vi "运维调试_五参数.vi"(11 "编号":string) -> ()   [LabVIEW 2016, in "斯坦道多参数.lvlib"]
uses:
  <vilib>/Utility/miscctls.llb/LVPointTypeDef.ctl
  <vilib>/Plasmionique/MB Master/MB_Master/MB_Master.lvclass
  <vilib>/Utility/config.llb/NI_LVConfig.lvlib
panel:
  in  "滤波次数":dbl caption="滤波次数:"
  in  "校准选择":T1
  out "模块版本号":string
  out "权限等级":string
  in  "ORP探头选择":u16(ring) items=["YL型", "MQ型", "NAQ型"]
  in  "ORP启用":bool
  in  "水样测量时间":dbl caption="水样测量时间:"
  in  "自动断线重连":bool=TRUE
  in  "打开modbus":bool
  out "选项卡控件":enum32{"选项卡 1", "选项卡 2"}(tab)
  in  "VISA资源名称":refnum<visa-resource-name> caption="串口"
  in  "IP":string="localhost" caption="IP:"
  in  "Port":u16=502 caption="Port:"
  in  "连接方式":u16(ring) items=["Modbus RTU", "Modbus TCP"]
  in  "密码锁":bool
  in  "藻密度探头选择":u16(ring) items=["YL型", "MQ型", "NAQ型"]
  in  "叶绿素a探头选择":u16(ring) items=["YL型", "MQ型", "NAQ型"]
  in  "浊度探头选择":u16(ring) items=["YL型", "MQ型", "NAQ型"]
  in  "电导率探头选择":u16(ring) items=["YL型", "MQ型", "NAQ型"]
  in  "DO探头选择":u16(ring) items=["YL型", "MQ型", "NAQ型"]
  in  "pH探头选择":u16(ring) items=["YL型", "MQ型", "NAQ型"]
  in  "设置页返回":bool
  in  "藻密度":bool
  in  "叶绿素a启用":bool
  in  "Temp":bool
  in  "Cond":bool
  in  "Turb":bool
  in  "DO":bool
  in  "pH":bool
  in  "周期设置":bool
  out "当前串口":string
  out "运行状态":enum16{"空闲", "水样测试", "标样核查"}(ring)
  in  "停止":bool
  in  "标样核查":bool
  in  "水样测试":bool
  in  "设置":bool
  in  "探头校正返回":bool
  in  "探头校正":bool
  out "检测值":T2
  # "请设置仪器连接方式"
  # "请选择要启用的参数"
  # "min"
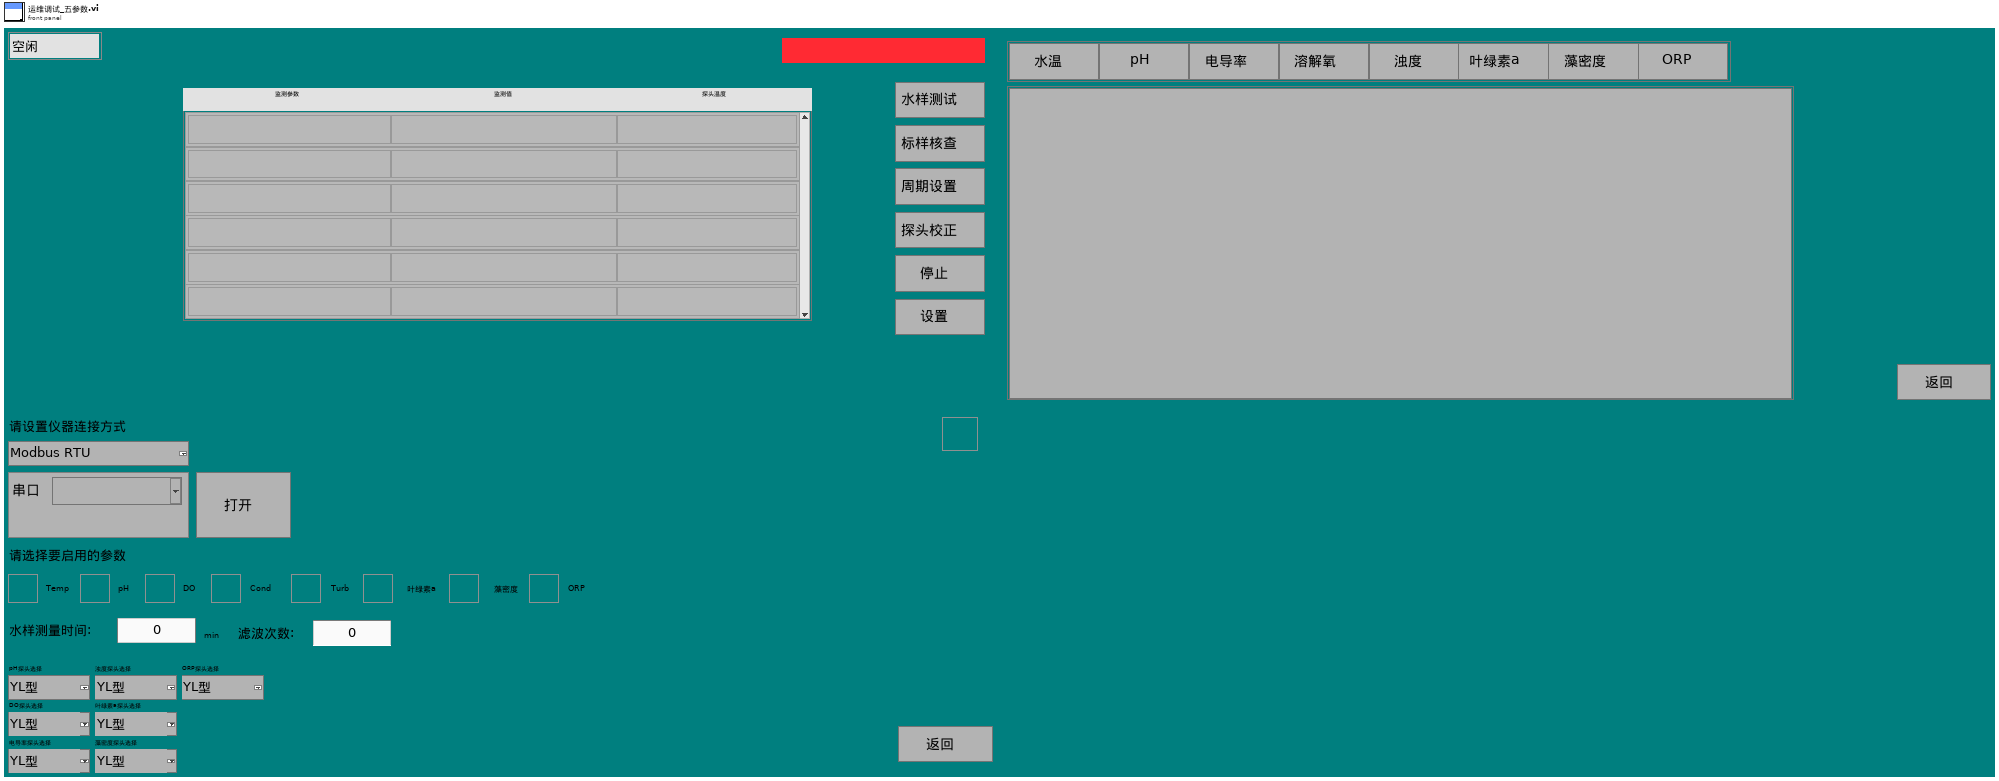
[diagram p1: front panel]
types:
  T1 = cluster{"水温校准":bool, "pH校准":bool, "电导率校准":bool, "溶解氧校准":bool, "浊度校准":bool, "叶绿素a校准":bool, "藻密度校准":bool, "ORP校准":bool}
  T2 = typedef "斯坦道多参数.lvlib/检测值.ctl" = cluster{"监测参数1":string, "浓度1":string, "探头温度1":string}[]
  T3 = typedef "LVPointTypeDef.ctl" = cluster{"Horizontal":i16, "Vertical":i16}
  T4 = enum8{"Enabled", "Disabled", "Disabled and Grayed Out"}
  T5 = cluster{"pH探头选择":u16, "DO探头选择":u16, "电导率探头选择":u16, "浊度探头选择":u16, "叶绿素a探头选择":u16, "蓝绿藻探头选择":u16, "orp探头选择":u16}
  T6 = cluster{"周期设置类型":enum16{"定点启动", "间隔启动"}, "定时功能启用":bool, "定时间隔":u32, "24H周期设置":bool[]}
  T7 = enum32{"Bad", "Idle", "Run top level", "Running"}
  T8 = typedef "LVDateTimeRec.ctl" = cluster{"秒数的小数部分":dbl, "秒":i32, "分":i32, "时":i32, "日":i32, "月":i32, "年":i32, "天数（周）":i32, "天数（年）":i32, "DST":i32}
  T9 = cluster{"Major":u16, "Minor":u16, "Fix":u16, "Build":u16}
  T10 = cluster{"监测参数1":string, "浓度1":string, "探头温度1":string}[]
  T11 = cluster{"温度测量值":sgl, "DO%":sgl, "DOmg/L":sgl, "温度偏移修正值":sgl}
  T12 = typedef "NI_LVConfig.lvlib/Config Data RefNum.ctl" = refnum<k1>
  T13 = cluster{"pH校准VI引用句柄":refnum<vi>, "DO校准VI引用句柄":refnum<vi>, "COND校准VI引用句柄":refnum<vi>, "TURB校准VI引用句柄":refnum<vi>, "CHLA校准VI引用句柄":refnum<vi>, "BGA校准VI引用句柄":refnum<vi>, "ORP校准VI引用句柄":refnum<vi>}
  T14 = cluster{"数据保存间隔":dbl, "水温标样值":dbl, "pH标样值":dbl, "溶解氧标样值":dbl, "电导率标样值":dbl, "浊度标样值":dbl}
  T15 = cluster{"baud rate (bps)":u32, "stop bits":u16, "parity":u16, "flow control":u16, "timeout":u32, "retries":i32}
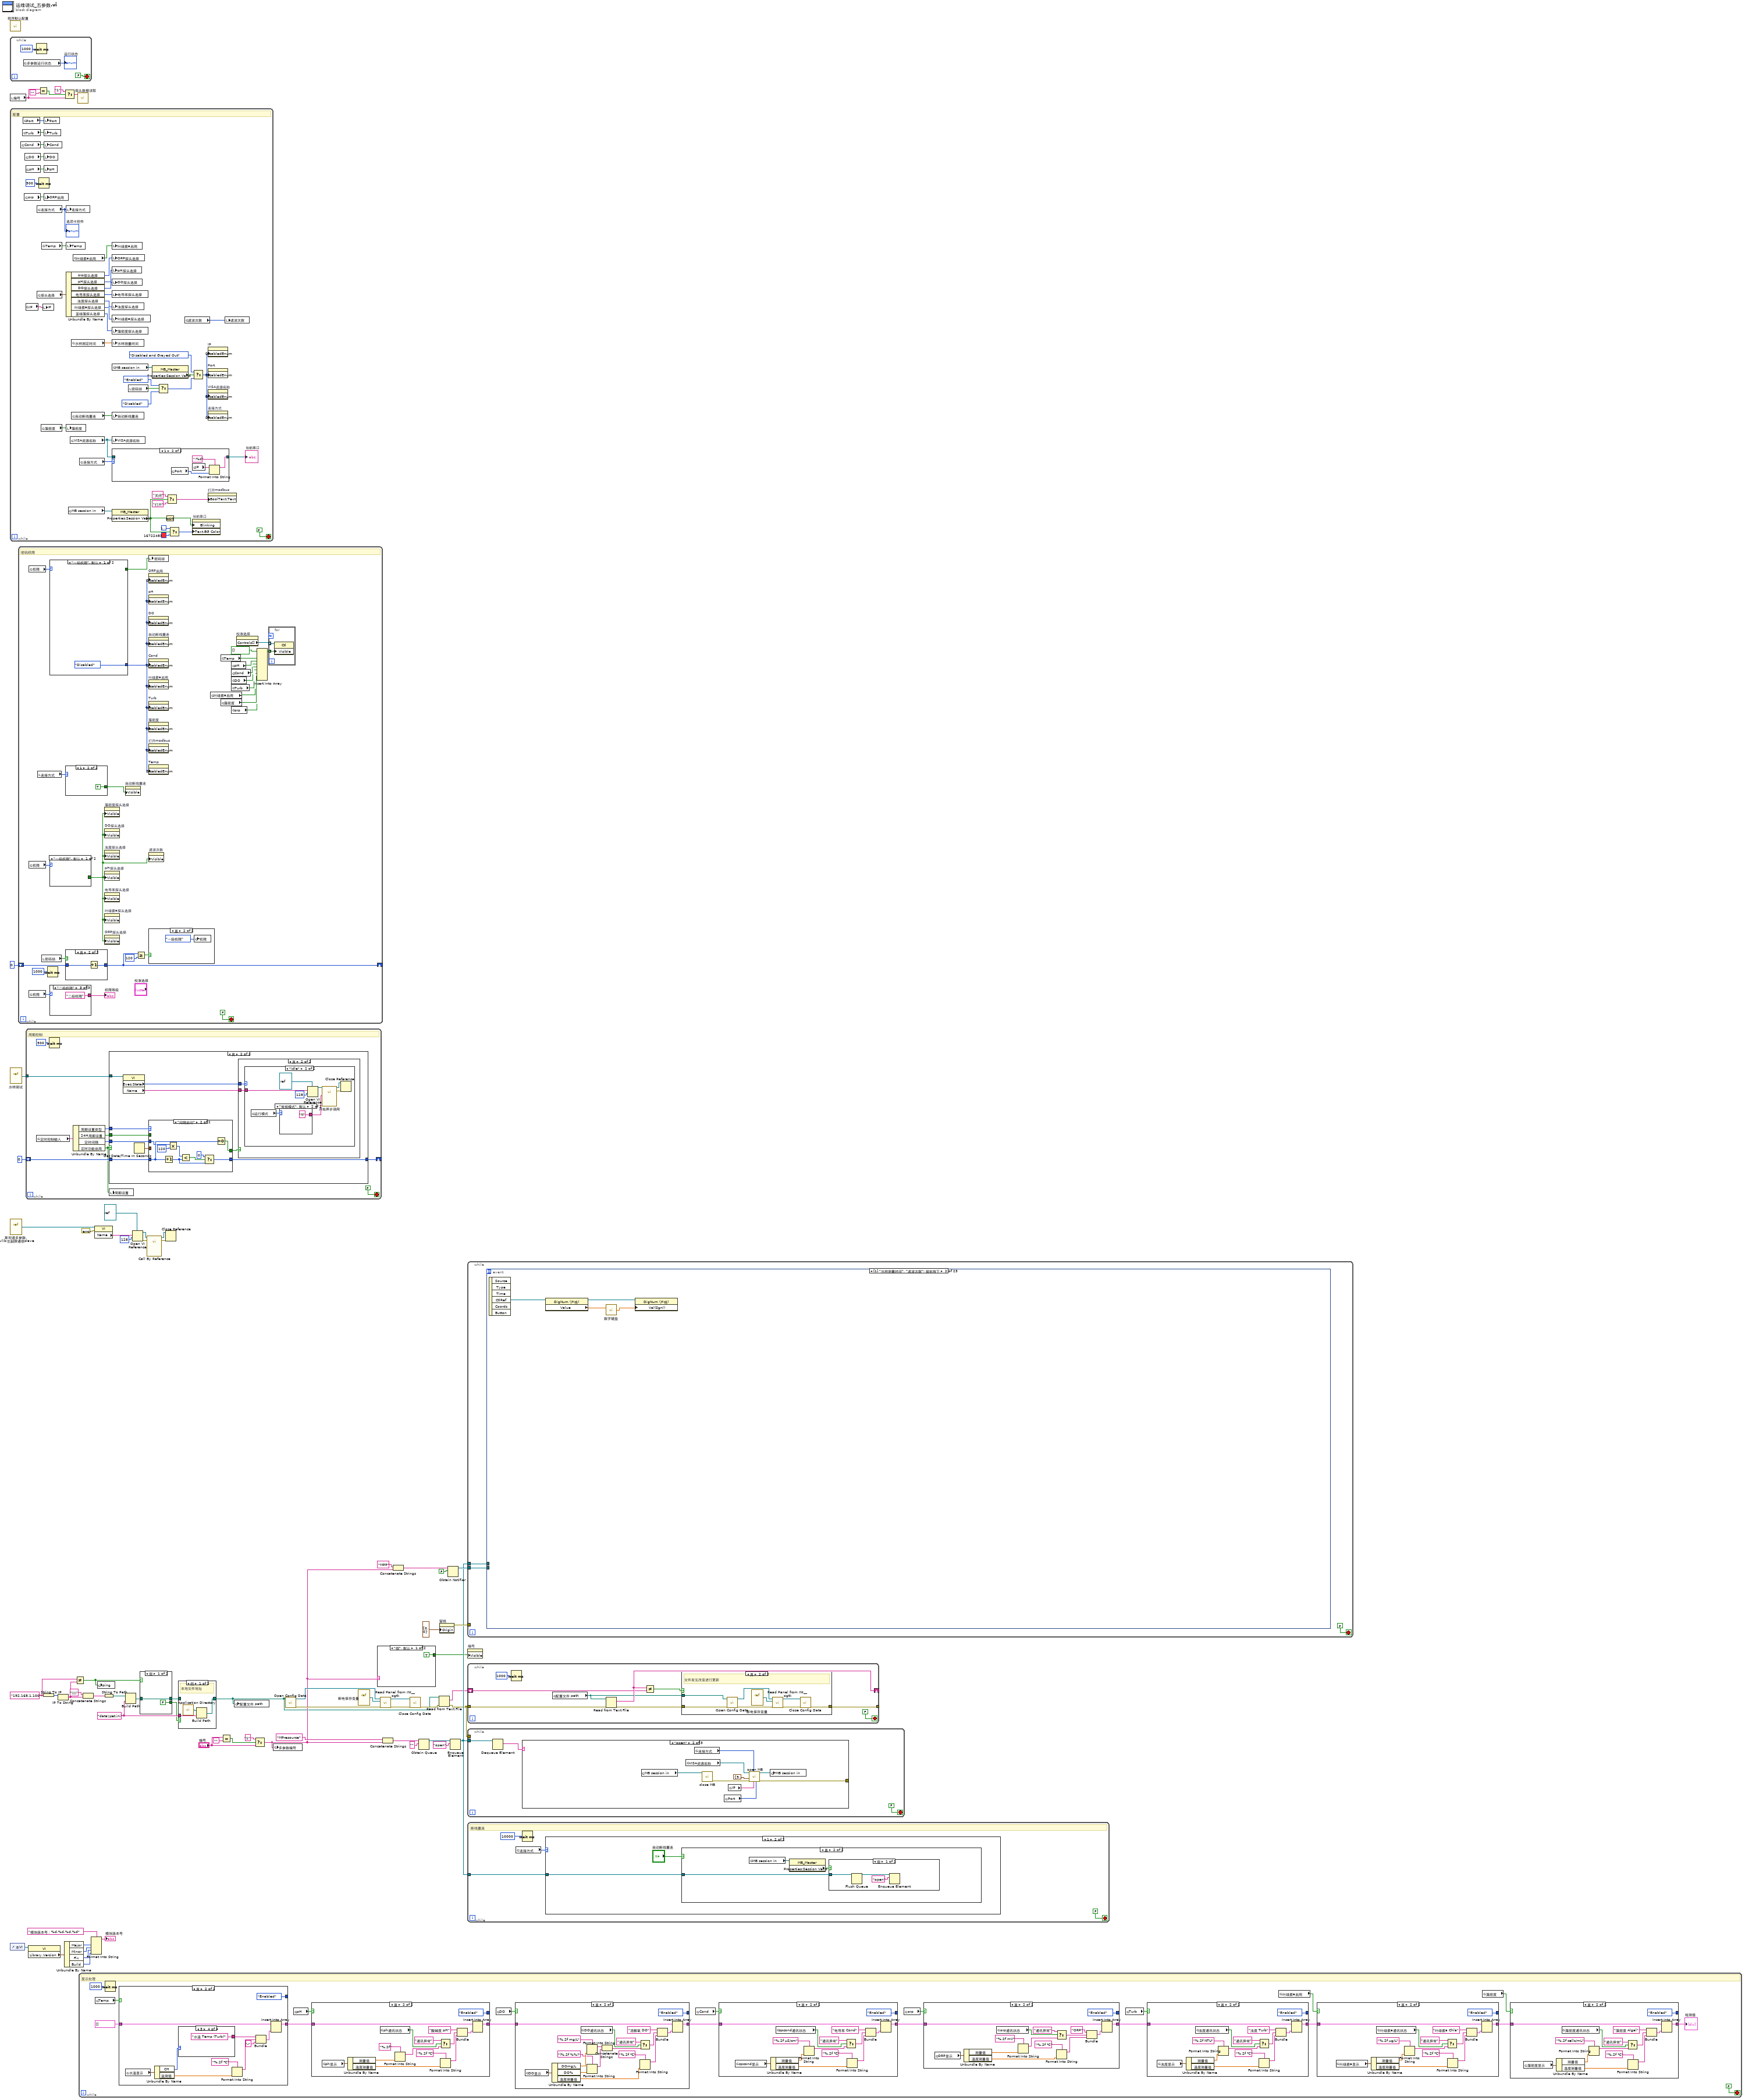
[diagram p0: block diagram]
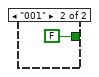
[diagram p2: hidden frame]
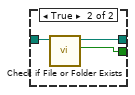
[diagram p4: hidden frame]
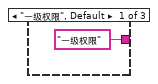
[diagram p12: hidden frame]
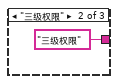
[diagram p13: hidden frame]
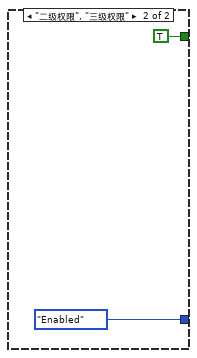
[diagram p14: hidden frame]
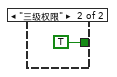
[diagram p15: hidden frame]
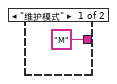
[diagram p19: hidden frame]
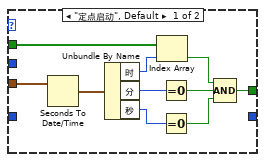
[diagram p20: hidden frame]
diagram:
  w34 = "data\\set.ini" ("名称或相对路径")
  w26 = "192.168.1.100" ("名称")
  n1 = call "程序默认配置.vi"() -> ()  [unwired: 11 in, 1 out]
  n2 = while {
    stop <- FALSE stop-if-true
    n3 = global read "多参数全局变量.vi" "多参数运行状态"() -> (→"运行状态":u16)
    n4 = Wait (ms)(milliseconds to wait=u32 1000 ("等待时间（毫秒）")) -> ()  [unwired: 1 out]
  }
  n5 = local read "编号"() -> (w6:string)
  n6 = while {
    stop <- FALSE stop-if-true
    # "配置"
    n7 = global read "断电保存变量.vi" "Cond"() -> (w106:bool)
    n8 = global read "断电保存变量.vi" "Turb"() -> (w105:bool)
    n9 = global read "断电保存变量.vi" "Port"() -> (w84:u16)
    n10 = global read "断电保存变量.vi" "orp"() -> (w69:bool)
    n11 = global read "断电保存变量.vi" "DO"() -> (w107:bool)
    n12 = global read "断电保存变量.vi" "pH"() -> (w108:bool)
    n13 = global read "断电保存变量.vi" "IP"() -> (w85:string)
    n14 = global read "断电保存变量.vi" "连接方式"() -> (w77:u16)
    "选项卡控件" <- w77
    n15 = global read "断电保存变量.vi" "探头选择"() -> (w95:T5)
    n16 = Wait (ms)(milliseconds to wait=u32 500 ("等待时间（毫秒）")) -> ()  [unwired: 1 out]
    n17 = global read "断电保存变量.vi" "藻密度"() -> (w103:bool)
    n18 = global read "断电保存变量.vi" "Temp"() -> (w109:bool)
    n19 = local write "IP"(w85) -> ()
    n20 = local write "Port"(w84) -> ()
    n21 = local write "Turb"(w105) -> ()
    n22 = local write "Cond"(w106) -> ()
    n23 = local write "DO"(w107) -> ()
    n24 = local write "pH"(w108) -> ()
    n25 = local write "ORP启用"(w69) -> ()
    n26 = local write "连接方式"(w77) -> ()
    n27 = local write "Temp"(w109) -> ()
    n28 = Unbundle By Name(w95) -> ("orp探头选择"=w68:u16, "pH探头选择"=w78:u16, "DO探头选择"=w94:u16, "电导率探头选择"=w93:u16, "浊度探头选择"=w92:u16, "叶绿素a探头选择"=w91:u16, "蓝绿藻探头选择"=w90:u16)
    n29 = local write "藻密度"(w103) -> ()
    n30 = global read "多参数全局变量.vi" "MB session in"() -> (w99:refnum<class "MB_Master.lvclass">)
    n31 = global read "断电保存变量.vi" "VISA资源名称"() -> (w81:refnum<visa-resource-name>)
    n32 = global read "断电保存变量.vi" "水样测定时间"() -> (w71:dbl)
    n33 = global read "断电保存变量.vi" "自动断线重连"() -> (w72:bool)
    n34 = global read "断电保存变量.vi" "叶绿素a启用"() -> (w104:bool)
    n35 = global read "断电保存变量.vi" "连接方式"() -> (w82:u16)
    n36 = local write "叶绿素a启用"(w104) -> ()
    n37 = local write "ORP探头选择"(w68) -> ()
    n38 = local write "pH探头选择"(w78) -> ()
    n39 = local write "DO探头选择"(w94) -> ()
    n40 = local write "电导率探头选择"(w93) -> ()
    n41 = local write "浊度探头选择"(w92) -> ()
    n42 = local write "叶绿素a探头选择"(w91) -> ()
    n43 = local write "藻密度探头选择"(w90) -> ()
    n44 = local write "水样测量时间"(w71) -> ()
    n45 = global read "多参数全局变量.vi" "MB session in"() -> (w102:refnum<class "MB_Master.lvclass">)
    n46 = local write "自动断线重连"(w72) -> ()
    n47 = local write "VISA资源名称"(w81) -> ()
    n48 = case shown="1" w82 {
      tunnel: w81 -> [w111 _]
      tunnel: [w111 w112] -> w80
      frame 0, Default {
      }
      frame 1 {
        n49 = global read "断电保存变量.vi" "Port"() -> (w113:u16)
        n50 = global read "断电保存变量.vi" "IP"() -> (w115:string)
        n51 = Format Into String(format string=":%d" ("格式字符串"), initial string=w115, w113) -> (resulting string=w112:string)  [unwired: 1 in, 1 out]
      }
    }
    "当前串口" <- w80
    n52 = property class="MB_Master"(reference=w99) -> ("Properties:Session Valid"=w76:bool)  [unwired: 1 in, 2 out]
    n53 = local read "密码锁"() -> (w89:bool)
    n54 = property class="MB_Master"(reference=w102) -> ("Properties:Session Valid"=w101:bool)  [unwired: 1 in, 2 out]
    n55 = Select(t=T4."Enabled" ("f"), s=w89, f=T4."Disabled") -> (s? t:f=w87:T4)
    n56 = Not(x=w76) -> (.not. x?=w79:bool)
    n57 = Select(t="关闭" ("布尔文本.文本"), s=w76, f="打开" ("布尔文本.文本")) -> (s? t:f=w96:string)
    n58 = Select(t=u32 16777216, s=w76, f=u32 16722483) -> (s? t:f=w73:u32)
    n59 = global read "断电保存变量.vi" "滤波次数"() -> (w67:u32)
    n60 = property on="当前串口" class="Str"("Blinking"=w79, "Text.BG Color"=w73) -> ()  [unwired: 2 in, 2 out]
    n61 = Select(t=T4."Disabled and Grayed Out" ("禁用"), s=w101, f=w87) -> (s? t:f=w83:T4)
    n62 = property on="IP" class="Str"("DisabledEnum"=w83) -> ()  [unwired: 2 in, 2 out]
    n63 = property on="Port" class="DigNum (严格)"("DisabledEnum"=w83) -> ()  [unwired: 2 in, 2 out]
    n64 = property on="VISA资源名称" class="VISAName"("DisabledEnum"=w83) -> ()  [unwired: 2 in, 2 out]
    n65 = property on="连接方式" class="Ring (严格)"("DisabledEnum"=w83) -> ()  [unwired: 2 in, 2 out]
    n66 = property on="打开modbus" class="Bool"("BoolText.Text"=w96) -> ()  [unwired: 2 in, 2 out]
    n67 = local write "滤波次数"(w67) -> ()
  }
  n68 = vi-ref "水样测试.vi"() -> (w53:refnum<vi>)
  n69 = vi-ref "斯坦道多参数.lvlib:主副屏通信slave.vi"() -> (w35:refnum<vi>)
  n70 = control-ref of="本VI"() -> (w22:refnum<vi>)
  n71 = while {
    shift-right: [w138] -> _
    shift-left: u32 0 ("等待时间（毫秒）") -> [w139]
    stop <- FALSE stop-if-true
    # "密码权限"
    n72 = global read "多参数全局变量.vi" "权限"() -> (w129:enum16{"一级权限", "二级权限", "三级权限"})
    n73 = global read "多参数全局变量.vi" "权限"() -> (w130:enum16{"一级权限", "二级权限", "三级权限"})
    n74 = global read "多参数全局变量.vi" "权限"() -> (w131:enum16{"一级权限", "二级权限", "三级权限"})
    n75 = local read "连接方式"() -> (w135:u16)
    n76 = local read "密码锁"() -> (w140:bool)
    n77 = Wait (ms)(milliseconds to wait=u32 1000 ("等待时间（毫秒）")) -> ()  [unwired: 1 out]
    n78 = case shown="\"一级权限\", 默认" w129 {
      tunnel: [T4."Disabled" ("禁用") T4."Enabled" ("禁用")] -> w133
      tunnel: [_ TRUE ("可见")] -> w128
      frame "一级权限", Default {
      }
      frame "二级权限", "三级权限" {
      }
    }
    n79 = case shown="\"一级权限\", 默认" w130 {
      tunnel: [_ TRUE ("可见")] -> w116
      frame "一级权限", Default {
      }
      frame "三级权限" {
      }
    }
    n80 = case shown="\"二级权限\"" w131 {
      tunnel: ["一级权限" ("权限等级") "三级权限" ("权限等级") "二级权限" ("权限等级")] -> w132
      frame "一级权限", Default {
      }
      frame "三级权限" {
      }
      frame "二级权限" {
      }
    }
    "权限等级" <- w132
    n81 = case shown="1" w135 {
      tunnel: [_ TRUE ("可见")] -> w134
      frame 0, Default {
      }
      frame 1 {
      }
    }
    n82 = case shown="真" w140 {
      tunnel: w139 -> [_ w148]
      tunnel: [_ w147] -> w138
      frame False {
      }
      frame True {
        n83 = Increment(x=w148) -> (x+1=w147:u32)
      }
    }
    n84 = property on="藻密度探头选择" class="Ring (严格)"("Visible"=w116) -> ()  [unwired: 2 in, 2 out]
    n85 = property on="DO探头选择" class="Ring (严格)"("Visible"=w116) -> ()  [unwired: 2 in, 2 out]
    n86 = property on="浊度探头选择" class="Ring (严格)"("Visible"=w116) -> ()  [unwired: 2 in, 2 out]
    n87 = property on="pH探头选择" class="Ring (严格)"("Visible"=w116) -> ()  [unwired: 2 in, 2 out]
    n88 = property on="电导率探头选择" class="Ring (严格)"("Visible"=w116) -> ()  [unwired: 2 in, 2 out]
    n89 = property on="叶绿素a探头选择" class="Ring (严格)"("Visible"=w116) -> ()  [unwired: 2 in, 2 out]
    n90 = property on="ORP探头选择" class="Ring (严格)"("Visible"=w116) -> ()  [unwired: 2 in, 2 out]
    n91 = property on="自动断线重连" class="Bool (严格)"("Visible"=w134) -> ()  [unwired: 2 in, 2 out]
    n92 = Greater Or Equal?(x=w138, y=u32 120) -> (x >= y?=w136:bool)
    n93 = local write "密码锁"(w128) -> ()
    n94 = property on="ORP启用" class="Bool (严格)"("DisabledEnum"=w133) -> ()  [unwired: 2 in, 2 out]
    n95 = property on="pH" class="Bool (严格)"("DisabledEnum"=w133) -> ()  [unwired: 2 in, 2 out]
    n96 = property on="DO" class="Bool (严格)"("DisabledEnum"=w133) -> ()  [unwired: 2 in, 2 out]
    n97 = property on="自动断线重连" class="Bool (严格)"("DisabledEnum"=w133) -> ()  [unwired: 2 in, 2 out]
    n98 = property on="Cond" class="Bool (严格)"("DisabledEnum"=w133) -> ()  [unwired: 2 in, 2 out]
    n99 = property on="叶绿素a启用" class="Bool (严格)"("DisabledEnum"=w133) -> ()  [unwired: 2 in, 2 out]
    n100 = property on="Turb" class="Bool (严格)"("DisabledEnum"=w133) -> ()  [unwired: 2 in, 2 out]
    n101 = property on="藻密度" class="Bool (严格)"("DisabledEnum"=w133) -> ()  [unwired: 2 in, 2 out]
    n102 = property on="打开modbus" class="Bool"("DisabledEnum"=w133) -> ()  [unwired: 2 in, 2 out]
    n103 = property on="Temp" class="Bool (严格)"("DisabledEnum"=w133) -> ()  [unwired: 2 in, 2 out]
    n104 = case shown="真" w136 {
      frame False {
      }
      frame True {
        n105 = global write "多参数全局变量.vi" "权限"(enum16{"一级权限", "二级权限", "三级权限"}."一级权限" ("权限")) -> ()
      }
    }
    n106 = property on="滤波次数" class="DigNum (严格)"("Visible"=w116) -> ()  [unwired: 2 in, 2 out]
    n107 = global read "断电保存变量.vi" "叶绿素a启用"() -> (w120:bool)
    n108 = global read "断电保存变量.vi" "Temp"() -> (w126:bool)
    n109 = global read "断电保存变量.vi" "藻密度"() -> (w119:bool)
    n110 = global read "断电保存变量.vi" "pH"() -> (w124:bool)
    n111 = global read "断电保存变量.vi" "Cond"() -> (w123:bool)
    n112 = global read "断电保存变量.vi" "DO"() -> (w122:bool)
    n113 = global read "断电保存变量.vi" "Turb"() -> (w121:bool)
    n114 = global read "断电保存变量.vi" "orp"() -> (w118:bool)
    n115 = property on="校准选择" class="Clust"() -> ("Controls[]"=w127:refnum<vi>[])  [unwired: 2 in, 2 out]
    n116 = Insert Into Array(array=bool[] [] ("数组"), new element #1=w126, new element #2=w124, new element #3=w123, new element #4=w122, new element #5=w121, new element #6=w120, new element #7=w119, new element #8=w118) -> (w117:bool[])  [unwired: 1 in]
    n117 = for {
      tunnel: w127 -> [w144] mode=indexing
      tunnel: w117 -> [w143] mode=indexing
      n118 = property class="Ctl"(reference=w144, "Visible"=w143) -> ()  [unwired: 1 in, 2 out]
    }
  }
  n119 = while {
    tunnel: w53 -> [w158]
    shift-right: [w157] -> _
    shift-left: u32 0 ("等待时间（毫秒）") -> [w159]
    stop <- FALSE stop-if-true
    # "周期控制"
    n120 = global read "断电保存变量.vi" "定时控制输入"() -> (w161:T6)
    n121 = Wait (ms)(milliseconds to wait=u32 500 ("等待时间（毫秒）")) -> ()  [unwired: 1 out]
    n122 = Unbundle By Name(w161) -> ("周期设置类型"=w163:enum16{"定点启动", "间隔启动"}, "24H周期设置"=w162:bool[], "定时间隔"=w160:u32, "定时功能启用"=w156:bool)
    n123 = case shown="真" w156 {
      tunnel: w163 -> [_ w174]
      tunnel: w162 -> [_ w173]
      tunnel: w160 -> [_ w171]
      tunnel: w159 -> [_ w167]
      tunnel: w158 -> [_ w170]
      tunnel: [_ w166] -> w157
      frame False {
      }
      frame True {
        n124 = property class="VI"(reference=w170) -> ("Exec.State"=w168:T7, "Name"=w169:string)  [unwired: 1 in, 2 out]
        n125 = Get Date/Time In Seconds() -> (seconds since 1Jan1904=w175:timestamp)
        n126 = case shown="\"间隔启动\"" w174 {
          tunnel: w175 -> [w197 _]
          tunnel: w173 -> [w194 _]
          tunnel: [w188 w205] -> w172
          tunnel: w171 -> [_ w204]
          tunnel: w167 -> [_ w206]
          tunnel: [_ w200] -> w166
          frame "定点启动", Default {
            n127 = Seconds To Date/Time(time stamp (now)=w197) -> (date time rec=w196:T8)  [unwired: 1 in]
            n128 = Unbundle By Name(w196) -> ("时"=w195:i32, "分"=w193:i32, "秒"=w192:i32)
            n129 = Index Array(array=w194, index=w195) -> (element=w191:bool)
            n130 = Equal To 0?(x=w193) -> (x = 0?=w190:bool)
            n131 = Equal To 0?(x=w192) -> (x = 0?=w189:bool)
            n132 = Compound Arithmetic op=AND ("复合运算")(w191, w190, w189) -> (w188:bool)
          }
          frame "间隔启动" {
            n133 = Increment(x=w206) -> (x+1=w199:u32)
            n134 = Multiply(x=w204, y=u32 120) -> (x*y=w198:u32)
            n135 = Less?(x=w198, y=w199) -> (x < y?=w202:bool)
            n136 = Select(t=u32 0 ("y"), s=w202, f=w199) -> (s? t:f=w200:u32)
            n137 = Equal To 0?(x=w206) -> (x = 0?=w205:bool)
          }
        }
        n138 = case shown="真" w172 {
          tunnel: w168 -> [_ w177]
          tunnel: w169 -> [_ w176]
          frame False {
          }
          frame True {
            n139 = case shown="\"Idle\"" w177 {
              tunnel: w176 -> [_ w182]
              frame "Bad", Default {
              }
              frame "Idle" {
                n140 = global read "多参数全局变量.vi" "运行模式"() -> (w180:enum16{"维护模式", "常规模式", "应急模式", "质控模式"})
                n141 = case shown="\"常规模式\", 默认" w180 {
                  tunnel: ["M" ("数据标记表") "N" ("数据标记表")] -> w179
                  frame "维护模式" {
                  }
                  frame "常规模式", Default {
                  }
                }
                n142 = Open VI Reference(type specifier VI Refnum (for type only)=refnum<vi> refnum, vi path=w182, options=128 ("选项")) -> (vi reference=w183:refnum<vi>)  [unwired: 3 in, 1 out]
                n143 = call-by-ref "开始异步调用"(reference=w183, "数据标记表"=w179) -> (reference out=w184:refnum<vi>, error out=w185:errorcluster)  [unwired: 12 in]
                n144 = Close Reference(reference=w184, error in (no error)=w185) -> ()  [unwired: 1 out]
              }
            }
          }
        }
      }
    }
    n145 = local write "周期设置"(w156) -> ()
  }
  n146 = property class="VI"(reference=w22) -> ("Library.Version"=w21:T9)  [unwired: 1 in, 2 out]
  n147 = Equal?(x=w6, y="") -> (x = y?=w8:bool)
  n148 = String To IP(1:w26) -> (0:w33:u32)
  n149 = IP To String(2:w33) -> (0:w30:string)  [unwired: 1 in]
  n150 = Unbundle By Name(w21) -> ("Major"=w19:u16, "Minor"=w18:u16, "Fix"=w17:u16, "Build"=w16:u16)
  n151 = Select(t="1", s=w8, f=w6) -> (s? t:f=w5:string)
  n152 = Not Equal?(x=w26, y=w30) -> (x != y?=w24:bool)
  n153 = call "探头数据读取.vi"("编号"=w5) -> ()  [unwired: 11 in]
  n154 = while {
    stop <- FALSE stop-if-true
    # "显示处理"
    n155 = global read "断电保存变量.vi" "Temp"() -> (w223:bool)
    n156 = Wait (ms)(milliseconds to wait=u32 1000 ("等待时间（毫秒）")) -> ()  [unwired: 1 out]
    n157 = case shown="真" w223 {
      tunnel: [w350 w355] -> w220
      tunnel: T10 [] ("数组") -> [w350 w356]
      tunnel: [T4."Disabled and Grayed Out" ("禁用") T4."Enabled" ("禁用")] -> _
      frame False {
      }
      frame True {
        n158 = global read "多参数全局变量.vi" "水温显示"() -> (w353:cluster{"CH":u16, "监测值":dbl, "温度偏移修正值":sgl})
        n159 = Unbundle By Name(w353) -> ("CH"=w352:u16, "监测值"=w351:dbl)
        n160 = case shown="3" w352 {
          tunnel: ["水温 Temp (pH)" ("监测参数1") "水温 Temp (Cond)" ("监测参数1") "水温 Temp (DO)" ("监测参数1") "水温 Temp (Turb)" ("监测参数1")] -> w360
          frame 0, Default {
          }
          frame 1 {
          }
          frame 2 {
          }
          frame 3 {
          }
        }
        n161 = Format Into String(format string="%.2f ℃" ("格式字符串"), w351) -> (resulting string=w359:string)  [unwired: 2 in, 1 out]
        n162 = Bundle("监测参数1"=w360, w359, "探头温度1"="-") -> (w357:cluster{"监测参数1":string, string, "探头温度1":string})  [unwired: 1 in]
        n163 = Insert Into Array(array=w356, new element=w357) -> (w355:T10)  [unwired: 1 in]
      }
    }
    n164 = global read "断电保存变量.vi" "pH"() -> (w221:bool)
    n165 = case shown="真" w221 {
      tunnel: [w333 w340] -> w218
      tunnel: w220 -> [w333 w342]
      tunnel: [T4."Disabled and Grayed Out" ("禁用") T4."Enabled" ("禁用")] -> _
      frame False {
      }
      frame True {
        n166 = global read "多参数全局变量.vi" "ph显示"() -> (w338:cluster{"温度测量值":sgl, "测量值":sgl, "温度偏移修正值":sgl})
        n167 = Unbundle By Name(w338) -> ("测量值"=w348:sgl, "温度测量值"=w346:sgl)
        n168 = global read "多参数全局变量.vi" "ph通讯状态"() -> (w336:bool)
        n169 = Format Into String(format string="%.2f" ("格式字符串"), w348) -> (resulting string=w335:string)  [unwired: 2 in, 1 out]
        n170 = Select(t="通讯异常" ("格式字符串"), s=w336, f=w335) -> (s? t:f=w334:string)
        n171 = Format Into String(format string="%.2f ℃" ("格式字符串"), w346) -> (resulting string=w344:string)  [unwired: 2 in, 1 out]
        n172 = Bundle("监测参数2"="酸碱度 pH", "格式字符串"=w334, w344) -> (w341:cluster{"监测参数2":string, "格式字符串":string, string})  [unwired: 1 in]
        n173 = Insert Into Array(array=w342, new element=w341) -> (w340:T10)  [unwired: 1 in]
      }
    }
    n174 = global read "断电保存变量.vi" "DO"() -> (w219:bool)
    n175 = case shown="真" w219 {
      tunnel: [w312 w319] -> w215
      tunnel: w218 -> [w312 w320]
      tunnel: [T4."Disabled and Grayed Out" ("禁用") T4."Enabled" ("禁用")] -> _
      frame False {
      }
      frame True {
        n176 = global read "多参数全局变量.vi" "DO显示"() -> (w317:T11)
        n177 = Unbundle By Name(w317) -> ("DOmg/L"=w328:sgl, "DO%"=w326:sgl, "温度测量值"=w330:sgl)
        n178 = global read "多参数全局变量.vi" "DO通讯状态"() -> (w315:bool)
        n179 = Format Into String(format string="%.2f mg/L" ("格式字符串"), w328) -> (resulting string=w325:string)  [unwired: 2 in, 1 out]
        n180 = Format Into String(format string="(%.2f %%)" ("格式字符串"), w326) -> (resulting string=w324:string)  [unwired: 2 in, 1 out]
        n181 = Concatenate Strings(w325, w324) -> (w314:string)
        n182 = Select(t="通讯异常" ("格式字符串"), s=w315, f=w314) -> (s? t:f=w313:string)
        n183 = Format Into String(format string="%.2f ℃" ("格式字符串"), w330) -> (resulting string=w322:string)  [unwired: 2 in, 1 out]
        n184 = Bundle("监测参数2"="溶解氧 DO", "格式字符串"=w313, w322) -> (w321:cluster{"监测参数2":string, "格式字符串":string, string})  [unwired: 1 in]
        n185 = Insert Into Array(array=w320, new element=w321) -> (w319:T10)  [unwired: 1 in]
      }
    }
    n186 = global read "断电保存变量.vi" "Cond"() -> (w217:bool)
    n187 = case shown="真" w217 {
      tunnel: w215 -> [w295 w306]
      tunnel: [w295 w296] -> w207
      tunnel: [T4."Disabled and Grayed Out" ("禁用") T4."Enabled" ("禁用")] -> _
      frame False {
      }
      frame True {
        n188 = global read "多参数全局变量.vi" "spcond显示"() -> (w303:cluster{"温度测量值":sgl, "测量值":sgl, "温度偏移修正值":sgl})
        n189 = Unbundle By Name(w303) -> ("测量值"=w302:sgl, "温度测量值"=w301:sgl)
        n190 = global read "多参数全局变量.vi" "spcond通讯状态"() -> (w299:bool)
        n191 = Format Into String(format string="%.2f μS/cm" ("格式字符串"), w302) -> (resulting string=w298:string)  [unwired: 2 in, 1 out]
        n192 = Select(t="通讯异常" ("格式字符串"), s=w299, f=w298) -> (s? t:f=w297:string)
        n193 = Format Into String(format string="%.2f ℃" ("格式字符串"), w301) -> (resulting string=w307:string)  [unwired: 2 in, 1 out]
        n194 = Bundle("监测参数2"="电导率 Cond", "格式字符串"=w297, w307) -> (w305:cluster{"监测参数2":string, "格式字符串":string, string})  [unwired: 1 in]
        n195 = Insert Into Array(array=w306, new element=w305) -> (w296:T10)  [unwired: 1 in]
      }
    }
    n196 = global read "断电保存变量.vi" "orp"() -> (w209:bool)
    n197 = case shown="真" w209 {
      tunnel: w207 -> [w227 w238]
      tunnel: [w227 w236] -> w208
      tunnel: [T4."Disabled and Grayed Out" ("禁用") T4."Enabled" ("禁用")] -> _
      frame False {
      }
      frame True {
        n198 = global read "多参数全局变量.vi" "ORP显示"() -> (w234:cluster{"温度测量值":sgl, "测量值":sgl, "温度偏移修正值":sgl})
        n199 = Unbundle By Name(w234) -> ("测量值"=w233:sgl, "温度测量值"=w232:sgl)
        n200 = global read "多参数全局变量.vi" "orp通讯状态"() -> (w230:bool)
        n201 = Format Into String(format string="%.2f mV" ("格式字符串"), w233) -> (resulting string=w229:string)  [unwired: 2 in, 1 out]
        n202 = Select(t="通讯异常" ("格式字符串"), s=w230, f=w229) -> (s? t:f=w228:string)
        n203 = Format Into String(format string="%.2f ℃" ("格式字符串"), w232) -> (resulting string=w239:string)  [unwired: 2 in, 1 out]
        n204 = Bundle("监测参数2"="ORP", "格式字符串"=w228, w239) -> (w237:cluster{"监测参数2":string, "格式字符串":string, string})  [unwired: 1 in]
        n205 = Insert Into Array(array=w238, new element=w237) -> (w236:T10)  [unwired: 1 in]
      }
    }
    n206 = global read "断电保存变量.vi" "Turb"() -> (w216:bool)
    n207 = case shown="真" w216 {
      tunnel: w208 -> [w278 w289]
      tunnel: [w278 w287] -> w214
      tunnel: [T4."Disabled and Grayed Out" ("禁用") T4."Enabled" ("禁用")] -> _
      frame False {
      }
      frame True {
        n208 = global read "多参数全局变量.vi" "浊度显示"() -> (w285:cluster{"温度测量值":sgl, "测量值":sgl, "温度偏移修正值":sgl})
        n209 = Unbundle By Name(w285) -> ("测量值"=w284:sgl, "温度测量值"=w283:sgl)
        n210 = global read "多参数全局变量.vi" "浊度通讯状态"() -> (w281:bool)
        n211 = Format Into String(format string="%.2f NTU" ("格式字符串"), w284) -> (resulting string=w280:string)  [unwired: 2 in, 1 out]
        n212 = Select(t="通讯异常" ("格式字符串"), s=w281, f=w280) -> (s? t:f=w279:string)
        n213 = Format Into String(format string="%.2f ℃" ("格式字符串"), w283) -> (resulting string=w291:string)  [unwired: 2 in, 1 out]
        n214 = Bundle("监测参数2"="浊度 Turb", "格式字符串"=w279, w291) -> (w288:cluster{"监测参数2":string, "格式字符串":string, string})  [unwired: 1 in]
        n215 = Insert Into Array(array=w289, new element=w288) -> (w287:T10)  [unwired: 1 in]
      }
    }
    n216 = global read "断电保存变量.vi" "叶绿素a启用"() -> (w213:bool)
    n217 = case shown="真" w213 {
      tunnel: w214 -> [w261 w272]
      tunnel: [w261 w270] -> w211
      tunnel: [T4."Disabled and Grayed Out" ("禁用") T4."Enabled" ("禁用")] -> _
      frame False {
      }
      frame True {
        n218 = global read "多参数全局变量.vi" "叶绿素a显示"() -> (w266:cluster{"温度测量值":sgl, "测量值":sgl, "温度偏移修正值":sgl})
        n219 = Unbundle By Name(w266) -> ("测量值"=w269:sgl, "温度测量值"=w268:sgl)
        n220 = global read "多参数全局变量.vi" "叶绿素a通讯状态"() -> (w264:bool)
        n221 = Format Into String(format string="%.2f μg/L" ("格式字符串"), w269) -> (resulting string=w263:string)  [unwired: 2 in, 1 out]
        n222 = Select(t="通讯异常" ("格式字符串"), s=w264, f=w263) -> (s? t:f=w262:string)
        n223 = Format Into String(format string="%.2f ℃" ("格式字符串"), w268) -> (resulting string=w274:string)  [unwired: 2 in, 1 out]
        n224 = Bundle("监测参数2"="叶绿素a Chla", "格式字符串"=w262, w274) -> (w271:cluster{"监测参数2":string, "格式字符串":string, string})  [unwired: 1 in]
        n225 = Insert Into Array(array=w272, new element=w271) -> (w270:T10)  [unwired: 1 in]
      }
    }
    n226 = global read "断电保存变量.vi" "藻密度"() -> (w212:bool)
    n227 = case shown="真" w212 {
      tunnel: w211 -> [w244 w255]
      tunnel: [w244 w253] -> w210
      tunnel: [T4."Disabled and Grayed Out" ("禁用") T4."Enabled" ("禁用")] -> _
      frame False {
      }
      frame True {
        n228 = global read "多参数全局变量.vi" "藻密度显示"() -> (w249:cluster{"温度测量值":sgl, "测量值":sgl, "温度偏移修正值":sgl})
        n229 = Unbundle By Name(w249) -> ("测量值"=w252:sgl, "温度测量值"=w251:sgl)
        n230 = global read "多参数全局变量.vi" "藻密度通讯状态"() -> (w247:bool)
        n231 = Format Into String(format string="%.2f cells/mL" ("格式字符串"), w252) -> (resulting string=w246:string)  [unwired: 2 in, 1 out]
        n232 = Select(t="通讯异常" ("格式字符串"), s=w247, f=w246) -> (s? t:f=w245:string)
        n233 = Format Into String(format string="%.2f ℃" ("格式字符串"), w251) -> (resulting string=w257:string)  [unwired: 2 in, 1 out]
        n234 = Bundle("监测参数2"="藻密度 Algal", "格式字符串"=w245, w257) -> (w254:cluster{"监测参数2":string, "格式字符串":string, string})  [unwired: 1 in]
        n235 = Insert Into Array(array=w255, new element=w254) -> (w253:T10)  [unwired: 1 in]
      }
    }
    "检测值" <- w210
  }
  n236 = Concatenate Strings("\\\\" ("字符串"), w30) -> (w31:string)
  n237 = Format Into String(format string="模块版本号：%d.%d.%d.%d" ("格式字符串"), w19, w18, w17, w16) -> (resulting string=→"模块版本号":string)  [unwired: 2 in, 1 out]
  n238 = property class="VI"(reference=w35, error in=errorcluster {"status"=FALSE, "code"=0, "source"=""} ("错误输出")) -> ("Name"=w36:string)  [unwired: 2 out]
  n239 = global write "多参数全局变量.vi" "ping"(w24) -> ()
  n240 = String To Path(string=w31) -> (path=w25:path)
  n241 = Build Path(base path=w25, name or relative path=w34) -> (appended path=w29:path)
  n242 = Open VI Reference(type specifier VI Refnum (for type only)=refnum<vi> refnum, vi path=w36, options=128 ("选项")) -> (vi reference=w38:refnum<vi>, error out=w40:errorcluster)  [unwired: 3 in]
  n243 = case shown="假" w24 {
    tunnel: w29 -> [w366 w370]
    tunnel: [w366 w369] -> w28
    tunnel: [FALSE w368] -> w27
    frame False {
    }
    frame True {
      n244 = call <vilib>:"Check if File or Folder Exists.vi"("path"=w370) -> ("file or folder exists?"=w368:bool, "dup path"=w369:path)  [unwired: 8 in, 1 out]
    }
  }
  n245 = call-by-ref "?"(reference=w38, error in=w40) -> (reference out=w42:refnum<vi>, error out=w41:errorcluster)  [unwired: 12 in]
  n246 = Close Reference(reference=w42, error in (no error)=w41) -> ()  [unwired: 1 out]
  n247 = case shown="假" w27 {
    tunnel: w28 -> [_ w374]
    tunnel: [w372 w374] -> w3
    tunnel: w34 -> [w371 _]
    frame False {
      # "本地文件地址"
      n248 = call <vilib>:"Application Directory.vi"() -> ("Application Directory"=w373:path)
      n249 = Build Path(base path=w373, name or relative path=w371) -> (appended path=w372:path)
    }
    frame True {
      # "网络共享地址"
    }
  }
  n250 = Equal?(x="编号", y="") -> (x = y?=w13:bool)
  n251 = global write "多参数全局变量.vi" "配置文件 path"(w3) -> ()
  n252 = Select(t="1", s=w13, f="编号") -> (s? t:f=w11:string)
  n253 = global write "多参数全局变量.vi" "多参数编号"(w11) -> ()
  n254 = call <vilib>:"Open Config Data.vi"("configuration file path"=w3) -> ("error out"=w47:errorcluster, "refnum"=w48:T12)  [unwired: 8 in, 1 out]
  n255 = vi-ref "断电保存变量.vi"() -> (w44:refnum<vi>)
  n256 = case shown="\"假\", 默认" w11 {
    tunnel: [TRUE ("可见") FALSE ("可见")] -> w23
    frame "假", Default {
    }
    frame "001" {
    }
  }
  n257 = call <userlib>:"Read Panel from INI__ogtk.vi"("error in (no error)"=w47, "VI ref"=w44, "refnum"=w48) -> ("error out"=w45:errorcluster, "refnum out"=w46:T12)  [unwired: 7 in]
  n258 = Concatenate Strings("MPresource" ("名称（未命名）"), w11) -> (w55:string)
  n259 = Concatenate Strings("MPP" ("名称（未命名）"), w11) -> (w56:string)
  n260 = call <vilib>:"Close Config Data.vi"("error in (no error)"=w45, "refnum"=w46) -> ("error out"=w4:errorcluster)  [unwired: 8 in, 1 out]
  n261 = Obtain Queue(name (unnamed)=w55, element data type="" ("名称（未命名）")) -> (queue out=w51:refnum<queue>)  [unwired: 3 in, 2 out]
  n262 = Read from Text File(file (use dialog)=w3, error in=w4) -> (text=w2:string, error out=w1:errorcluster)  [unwired: 2 in, 2 out]
  n263 = property on="窗格" class="Pane"("Origin"=T3 {"Horizontal"=0, "Vertical"=0} ("原点")) -> (error out=w63:errorcluster)  [unwired: 2 in, 1 out]
  n264 = Obtain Notifier(name (unnamed)=w56, notification data type=FALSE) -> (notifier out=w59:refnum<notifier>)  [unwired: 2 in, 2 out]
  n265 = Enqueue Element(queue=w51, element="open" ("元素")) -> (queue out=w50:refnum<queue>)  [unwired: 2 in, 2 out]
  n266 = while {
    tunnel: w63 -> [_]
    tunnel: w59 -> [w378]
    tunnel: w50 -> [w377]
    stop <- FALSE stop-if-true
    n267 = event shown="[1] \"水样测量时间\", \"滤波次数\": 鼠标按下" {
      selector: _ -> [_ _ _ _ _ _ _ _ _ _ _ _ _ _ _ _ _ _ _ _ _ _ _]
      dyn-events: _ -> [_ _ _ _ _ _ _ _ _ _ _ _ _ _ _ _ _ _ _ _ _ _ _]
      timeout: _ -> [_ _ _ _ _ _ _ _ _ _ _ _ _ _ _ _ _ _ _ _ _ _ _]
      tunnel: w378 -> [_ _ _ _ _ _ _ _ _ _ w483 _ _ _ _ _ _ _ _ _ _ _ _]
      tunnel: w377 -> [_ _ _ _ _ _ _ _ _ _ _ _ _ w501 _ _ _ _ _ _ _ _ _]
      event Timeout {
        n268 = event-data() -> ()  [unwired: 1 in, 3 out]
      }
      event "水样测量时间", "滤波次数": Mouse Down {
        n269 = event-data() -> ("CtlRef"=w380:refnum<vi>)  [unwired: 1 in, 5 out]
        n270 = property class="DigNum (严格)"(reference=w380) -> (reference out=w383:refnum<vi>, "Value"=w382:dbl)  [unwired: 1 in, 1 out]
        n271 = call "数字键盘.vi"("OldNumber"=w382) -> ("NewNumber"=w381:dbl)  [unwired: 1 in]
        n272 = property class="DigNum (严格)"(reference=w383, "Val(Sgnl)"=w381) -> ()  [unwired: 1 in, 2 out]
      }
      event "pH探头选择", "DO探头选择", "电导率探头选择", "浊度探头选择", "叶绿素a探头选择", "藻密度探头选择", "ORP探头选择": Value Change {
        n273 = event-data() -> ("CtlRef"=w384:refnum<vi>, "NewVal"=w385:u16)  [unwired: 1 in, 4 out]
        n274 = Two Button Dialog(message="请再次确认修改的型号是否与实际匹配，否则将导致通讯异常，并且此操作将终止所有正在校准的参数！" ("消息")) -> (T button?=w386:bool)  [unwired: 2 in]
        n275 = case shown="真" w386 {
          tunnel: w385 -> [_ w389]
          tunnel: w384 -> [_ w388]
          frame False {
          }
          frame True {
            n276 = flat-sequence {
              tunnel: w389 -> [w390]
              tunnel: w388 -> [w394]
              frame #0 {
                n277 = property class="Ring (严格)"(reference=w394) -> ("Label.Text"=w393:string)  [unwired: 1 in, 2 out]
                n278 = global read "断电保存变量.vi" "探头选择"() -> (w392:T5)
                n279 = global read "多参数全局变量.vi" "校准VI引用句柄"() -> (w395:T13)
                n280 = case shown="\"ORP探头选择\"" w393 {
                  tunnel: w392 -> [w397 w400 w403 w406 w409 w412 w415 w418]
                  tunnel: [w397 w399 w402 w405 w408 w411 w414 w417] -> w391
                  tunnel: w390 -> [_ w398 w401 w404 w407 w410 w413 w416]
                  frame Default {
                  }
                  frame "pH探头选择" {
                    n281 = Bundle By Name(cluster=w400, "pH探头选择"=w398) -> (w399:T5)
                  }
                  frame "电导率探头选择" {
                    n282 = Bundle By Name(cluster=w403, "电导率探头选择"=w401) -> (w402:T5)
                  }
                  frame "DO探头选择" {
                    n283 = Bundle By Name(cluster=w406, "DO探头选择"=w404) -> (w405:T5)
                  }
                  frame "浊度探头选择" {
                    n284 = Bundle By Name(cluster=w409, "浊度探头选择"=w407) -> (w408:T5)
                  }
                  frame "叶绿素a探头选择" {
                    n285 = Bundle By Name(cluster=w412, "叶绿素a探头选择"=w410) -> (w411:T5)
                  }
                  frame "蓝绿藻探头选择" {
                    n286 = Bundle By Name(cluster=w415, "蓝绿藻探头选择"=w413) -> (w414:T5)
                  }
                  frame "ORP探头选择" {
                    n287 = Bundle By Name(cluster=w418, "蓝绿藻探头选择"=w416) -> (w417:T5)
                  }
                }
                n288 = Cluster To Array(cluster=w395) -> (array=w396:refnum<vi>[])
                n289 = for {
                  tunnel: w396 -> [w420] mode=indexing
                  tunnel: [w419] -> _ mode=indexing
                  n290 = invoke class="VI" method="Abort VI"(reference=w420) -> (error out=w419:errorcluster)  [unwired: 2 in, 2 out]
                }
                n291 = global write "断电保存变量.vi" "探头选择"(w391) -> ()
              }
              frame #1 {
                n292 = call "配置文件保存.vi"() -> ()  [unwired: 12 in]
              }
            }
          }
        }
      }
      event "VISA资源名称", "pH", "DO", "Turb", "Cond", "Temp", "叶绿素a启用", "打开modbus", "藻密度", "连接方式", "自动断线重连", "ORP启用": Mouse Down {
        n293 = event-data() -> ()  [unwired: 1 in, 6 out]
        n294 = local read "密码锁"() -> (w421:bool)
        n295 = case shown="假" w421 {
          frame False {
            n296 = One Button Dialog(message="当前操作权限不足,请提升权限!!!" ("消息")) -> ()  [unwired: 1 in, 1 out]
          }
          frame True {
          }
        }
      }
      event "IP": Mouse Down {
        n297 = event-data() -> ("CtlRef"=w424:refnum<vi>)  [unwired: 1 in, 7 out]
        n298 = property on="IP" class="Str"() -> ("DisabledEnum"=w423:T4)  [unwired: 2 in, 2 out]
        n299 = case shown="\"Disabled and Grayed Out\"" w423 {
          tunnel: w424 -> [w428 _ _]
          frame "Enabled" {
            n300 = property class="Str"(reference=w428) -> (reference out=w427:refnum<vi>, "Value"=w426:string)  [unwired: 1 in, 1 out]
            n301 = call "字符键盘.vi"("Old String"=w426) -> ("String"=w425:string)  [unwired: 10 in]
            n302 = property class="Str"(reference=w427, "Val(Sgnl)"=w425) -> ()  [unwired: 1 in, 2 out]
          }
          frame "Disabled and Grayed Out" {
            n303 = One Button Dialog(message="关闭连接后才可设置!" ("消息")) -> ()  [unwired: 1 in, 1 out]
          }
          frame "Disabled", Default {
            n304 = One Button Dialog(message="当前操作权限不足,请提升权限!!!" ("消息")) -> ()  [unwired: 1 in, 1 out]
          }
        }
      }
      event "Port": Mouse Down {
        n305 = event-data() -> ("CtlRef"=w432:refnum<vi>)  [unwired: 1 in, 7 out]
        n306 = property on="Port" class="DigNum (严格)"() -> ("DisabledEnum"=w431:T4)  [unwired: 2 in, 2 out]
        n307 = case shown="\"Enabled\"" w431 {
          tunnel: w432 -> [w436 _ _]
          frame "Enabled" {
            n308 = property class="DigNum (严格)"(reference=w436) -> (reference out=w435:refnum<vi>, "Value"=w434:u16)  [unwired: 1 in, 1 out]
            n309 = call "数字键盘.vi"("OldNumber"=w434) -> ("NewNumber"=w433:dbl)  [unwired: 1 in]
            n310 = property class="DigNum (严格)"(reference=w435, "Val(Sgnl)"=w433) -> ()  [unwired: 1 in, 2 out]
          }
          frame "Disabled and Grayed Out" {
            n311 = One Button Dialog(message="关闭连接后才可设置!" ("消息")) -> ()  [unwired: 1 in, 1 out]
          }
          frame "Disabled", Default {
            n312 = One Button Dialog(message="当前操作权限不足,请提升权限!!!" ("消息")) -> ()  [unwired: 1 in, 1 out]
          }
        }
      }
      event "密码锁": Value Change {
        n313 = event-data() -> ("NewVal"=w439:bool)  [unwired: 1 in, 5 out]
        n314 = case shown="假" w439 {
          frame False {
            n315 = global write "多参数全局变量.vi" "权限"(enum16{"一级权限", "二级权限", "三级权限"}."一级权限" ("权限")) -> ()
          }
          frame True {
            n316 = call "数字键盘.vi"("显示样式"=u32 2) -> ("NewNumber"=w444:dbl)  [unwired: 1 in]
            n317 = case shown="23506" w444 {
              tunnel: ["密码错误,即将切换为一级权限!" ("Infoin") "密码正确,即将切换为二级权限!" ("Infoin") "密码正确,即将切换为三级权限!" ("Infoin")] -> w443
              tunnel: [u32 16711680 ("颜色盒") _ _] -> w442
              tunnel: [enum16{"一级权限", "二级权限", "三级权限"}."一级权限" ("权限") enum16{"一级权限", "二级权限", "三级权限"}."二级权限" ("权限") enum16{"一级权限", "二级权限", "三级权限"}."三级权限" ("权限")] -> w441
              frame 0, Default {
              }
              frame 666 {
              }
              frame 23506 {
              }
            }
            n318 = global write "多参数全局变量.vi" "权限"(w441) -> ()
            n319 = call "TimeLmtDialog.vi"("颜色盒"=w442, "Infoin"=w443) -> ()  [unwired: 10 in]
          }
        }
      }
      event "周期设置": Mouse Down {
        n320 = event-data() -> ()  [unwired: 1 in, 6 out]
        n321 = flat-sequence {
          frame #0 {
            n322 = global read "断电保存变量.vi" "定时控制输入"() -> (w454:T6)
            n323 = call "周期设置.vi"("定时控制输入"=w454) -> ("定时控制输出"=w453:T6)  [unwired: 10 in]
            n324 = global write "断电保存变量.vi" "定时控制输入"(w453) -> ()
          }
          frame #1 {
            n325 = call "配置文件保存.vi"() -> ()  [unwired: 12 in]
          }
        }
      }
      event "水样测试": Value Change {
        n326 = event-data() -> ()  [unwired: 1 in, 6 out]
        n327 = vi-ref "水样测试.vi"() -> (w457:refnum<vi>)
        n328 = property class="VI"(reference=w457) -> ("Name"=w461:string, "Exec.State"=w459:T7)  [unwired: 1 in, 2 out]
        n329 = Open VI Reference(type specifier VI Refnum (for type only)=refnum<vi> refnum, vi path=w461, options=128 ("选项")) -> (vi reference=w462:refnum<vi>)  [unwired: 3 in, 1 out]
        n330 = case shown="\"Idle\"" w459 {
          tunnel: [w463 w466] -> w458
          tunnel: w462 -> [w463 w465]
          tunnel: "hd" ("数据标记表") -> [_ w464]
          frame "Bad", Default {
          }
          frame "Idle" {
            n331 = call-by-ref "开始异步调用"(reference=w465, "数据标记表"=w464) -> (reference out=w466:refnum<vi>)  [unwired: 12 in, 1 out]
          }
        }
        n332 = Close Reference(reference=w458) -> ()  [unwired: 1 in, 1 out]
      }
      event "标样核查": Value Change {
        n333 = event-data() -> ()  [unwired: 1 in, 6 out]
        n334 = call "标样核查配置.vi"() -> ("确认输出"=w468:bool, "标样核查配置"=w467:T14)  [unwired: 10 in]
        n335 = case shown="真" w468 {
          tunnel: w467 -> [_ w470]
          frame False {
          }
          frame True {
            n336 = vi-ref "标样核查.vi"() -> (w471:refnum<vi>)
            n337 = property class="VI"(reference=w471) -> ("Name"=w475:string, "Exec.State"=w473:T7)  [unwired: 1 in, 2 out]
            n338 = Open VI Reference(type specifier VI Refnum (for type only)=refnum<vi> refnum, vi path=w475, options=128 ("选项")) -> (vi reference=w476:refnum<vi>)  [unwired: 3 in, 1 out]
            n339 = case shown="\"Idle\"" w473 {
              tunnel: [w477 w480] -> w472
              tunnel: w476 -> [w477 w479]
              tunnel: w470 -> [_ w478]
              frame "Bad", Default {
              }
              frame "Idle" {
                n340 = call-by-ref "开始异步调用"(reference=w479, "标样核查配置"=w478) -> (reference out=w480:refnum<vi>)  [unwired: 12 in, 1 out]
              }
            }
            n341 = Close Reference(reference=w472) -> ()  [unwired: 1 in, 1 out]
          }
        }
      }
      event "停止": Value Change {
        w481 = u16 3 items=["空闲", "水样测试", "标样核查", "停止"] ("主副屏同步启动")
        n342 = event-data() -> ()  [unwired: 1 in, 6 out]
        n343 = Send Notification(notification=TRUE ("通知"), notifier=w483) -> ()  [unwired: 1 in, 2 out]
        n344 = global write "多参数全局变量.vi" "主副屏同步启动"(w481) -> ()
      }
      event "设置": Value Change {
        n345 = event-data() -> ()  [unwired: 1 in, 6 out]
        n346 = property on="窗格" class="Pane"("Origin"=T3 {"Horizontal"=0, "Vertical"=628} ("原点")) -> ()  [unwired: 2 in, 2 out]
      }
      event "pH", "DO", "Turb", "Cond", "Temp", "叶绿素a启用", "藻密度", "VISA资源名称", "连接方式", "IP", "Port", "自动断线重连", "水样测量时间", "ORP启用", "滤波次数": Value Change {
        n347 = event-data() -> ()  [unwired: 1 in, 6 out]
        n348 = flat-sequence {
          frame #0 {
            n349 = global write "断电保存变量.vi" "Cond"("Cond") -> ()
            n350 = global write "断电保存变量.vi" "连接方式"("连接方式") -> ()
            n351 = global write "断电保存变量.vi" "orp"("ORP启用") -> ()
            n352 = global write "断电保存变量.vi" "pH"("pH") -> ()
            n353 = global write "断电保存变量.vi" "藻密度"("藻密度") -> ()
            n354 = global write "断电保存变量.vi" "Port"("Port") -> ()
            n355 = global write "断电保存变量.vi" "Temp"("Temp") -> ()
            n356 = global write "断电保存变量.vi" "Turb"("Turb") -> ()
            n357 = global write "断电保存变量.vi" "DO"("DO") -> ()
            n358 = global write "断电保存变量.vi" "IP"("IP") -> ()
            n359 = global write "断电保存变量.vi" "水样测定时间"("水样测量时间") -> ()
            n360 = global write "断电保存变量.vi" "VISA资源名称"("VISA资源名称") -> ()
            n361 = global write "断电保存变量.vi" "叶绿素a启用"("叶绿素a启用") -> ()
            n362 = local read "自动断线重连"() -> (w488:bool)
            n363 = global write "断电保存变量.vi" "滤波次数"("滤波次数") -> ()
            n364 = global write "断电保存变量.vi" "自动断线重连"(w488) -> ()
          }
          frame #1 {
            n365 = call "配置文件保存.vi"() -> ()  [unwired: 12 in]
          }
          frame #2 {
          }
        }
      }
      event "打开modbus": Value Change {
        n366 = event-data() -> ()  [unwired: 1 in, 6 out]
        n367 = global read "多参数全局变量.vi" "MB session in"() -> (w506:refnum<class "MB_Master.lvclass">)
        n368 = Flush Queue(queue=w501) -> (queue out=w500:refnum<queue>)  [unwired: 1 in, 2 out]
        n369 = property class="MB_Master"(reference=w506) -> ("Properties:Session Valid"=w505:bool)  [unwired: 1 in, 2 out]
        n370 = Select(t="close" ("元素"), s=w505, f="open" ("元素")) -> (s? t:f=w502:string)
        n371 = Enqueue Element(queue=w500, element=w502) -> ()  [unwired: 2 in, 3 out]
      }
      event "探头校正返回", "设置页返回": Value Change {
        n372 = event-data() -> ()  [unwired: 1 in, 6 out]
        n373 = property on="窗格" class="Pane"("Origin"=T3 {"Horizontal"=0, "Vertical"=0} ("原点")) -> ()  [unwired: 2 in, 2 out]
      }
      event "探头校正", "校准选择.水温校准": Value Change {
        n374 = event-data() -> ()  [unwired: 1 in, 6 out]
        n375 = property on="窗格" class="Pane"("Origin"=T3 {"Horizontal"=1656, "Vertical"=0} ("原点")) -> ()  [unwired: 2 in, 2 out]
        n376 = vi-ref "水温校准.vi"() -> (w508:refnum<vi>)
        n377 = property class="VI"(reference=w508) -> (reference out=w510:refnum<vi>, "Exec.State"=w509:T7)  [unwired: 1 in, 1 out]
        n378 = case shown="\"Bad\", 默认" w509 {
          tunnel: [w514 w516] -> w512
          tunnel: w510 -> [w514 w515]
          frame "Bad", Default {
          }
          frame "Idle" {
            n379 = invoke class="VI" method="Run VI"(reference=w515, "Wait until done"=FALSE ("结束前等待"), "Auto Dispose Ref"=FALSE ("自动销毁引用")) -> (reference out=w516:refnum<vi>)  [unwired: 2 in, 4 out]
          }
        }
        n380 = invoke on="探头校准子面板" class="SubPnl" method="Remove VI"() -> (error out=w511:errorcluster)  [unwired: 3 in, 2 out]
        n381 = invoke on="探头校准子面板" class="SubPnl" method="Insert VI"(error in=w511, "VI Ref"=w512) -> ()  [unwired: 2 in, 4 out]
      }
      event "校准选择.pH校准": Value Change {
        n382 = event-data() -> ()  [unwired: 1 in, 6 out]
        n383 = global read "断电保存变量.vi" "探头选择"() -> (w524:T5)
        n384 = Unbundle By Name(w524) -> ("pH探头选择"=w523:u16)
        n385 = case shown="2" w523 {
          tunnel: [w528 w529 w530] -> w522
          frame 0, Default {
            n386 = vi-ref "斯坦道多参数.lvlib:禹山pH校准.vi"() -> (w528:refnum<vi>)
          }
          frame 1 {
            n387 = vi-ref "斯坦道多参数.lvlib:pH电极校准.vi"() -> (w529:refnum<vi>)
          }
          frame 2 {
            n388 = vi-ref "斯坦道多参数.lvlib:纳清pH电极校准.vi"() -> (w530:refnum<vi>)
          }
        }
        n389 = property class="VI"(reference=w522) -> (reference out=w526:refnum<vi>, "Exec.State"=w525:T7)  [unwired: 1 in, 1 out]
        n390 = case shown="\"Bad\", 默认" w525 {
          tunnel: w526 -> [w531 w535]
          tunnel: [w531 w532] -> w520
          frame "Bad", Default {
          }
          frame "Idle" {
            n391 = invoke class="VI" method="Run VI"(reference=w535, "Wait until done"=FALSE ("结束前等待"), "Auto Dispose Ref"=FALSE ("自动销毁引用")) -> (reference out=w532:refnum<vi>)  [unwired: 2 in, 4 out]
          }
        }
        n392 = global read "多参数全局变量.vi" "校准VI引用句柄"() -> (w521:T13)
        n393 = invoke on="探头校准子面板" class="SubPnl" method="Remove VI"() -> (error out=w527:errorcluster)  [unwired: 3 in, 2 out]
        n394 = invoke on="探头校准子面板" class="SubPnl" method="Insert VI"(error in=w527, "VI Ref"=w520) -> ()  [unwired: 2 in, 4 out]
        n395 = Bundle By Name(cluster=w521, "pH校准VI引用句柄"=w520) -> (w519:T13)
        n396 = global write "多参数全局变量.vi" "校准VI引用句柄"(w519) -> ()
      }
      event "校准选择.电导率校准": Value Change {
        n397 = event-data() -> ()  [unwired: 1 in, 6 out]
        n398 = global read "断电保存变量.vi" "探头选择"() -> (w541:T5)
        n399 = Unbundle By Name(w541) -> ("电导率探头选择"=w540:u16)
        n400 = case shown="2" w540 {
          tunnel: [w545 w546 w547] -> w539
          frame 0, Default {
            n401 = vi-ref "斯坦道多参数.lvlib:禹山电导率校准.vi"() -> (w545:refnum<vi>)
          }
          frame 1 {
            n402 = vi-ref "斯坦道多参数.lvlib:电导率电极校准.vi"() -> (w546:refnum<vi>)
          }
          frame 2 {
            n403 = vi-ref "斯坦道多参数.lvlib:纳清电导率电极校准.vi"() -> (w547:refnum<vi>)
          }
        }
        n404 = property class="VI"(reference=w539) -> (reference out=w543:refnum<vi>, "Exec.State"=w542:T7)  [unwired: 1 in, 1 out]
        n405 = case shown="\"Bad\", 默认" w542 {
          tunnel: [w548 w550] -> w536
          tunnel: w543 -> [w548 w549]
          frame "Bad", Default {
          }
          frame "Idle" {
            n406 = invoke class="VI" method="Run VI"(reference=w549, "Wait until done"=FALSE ("结束前等待"), "Auto Dispose Ref"=FALSE ("自动销毁引用")) -> (reference out=w550:refnum<vi>)  [unwired: 2 in, 4 out]
          }
        }
        n407 = global read "多参数全局变量.vi" "校准VI引用句柄"() -> (w538:T13)
        n408 = invoke on="探头校准子面板" class="SubPnl" method="Remove VI"() -> (error out=w544:errorcluster)  [unwired: 3 in, 2 out]
        n409 = Bundle By Name(cluster=w538, "COND校准VI引用句柄"=w536) -> (w537:T13)
        n410 = invoke on="探头校准子面板" class="SubPnl" method="Insert VI"(error in=w544, "VI Ref"=w536) -> ()  [unwired: 2 in, 4 out]
        n411 = global write "多参数全局变量.vi" "校准VI引用句柄"(w537) -> ()
      }
      event "校准选择.溶解氧校准": Value Change {
        n412 = event-data() -> ()  [unwired: 1 in, 6 out]
        n413 = global read "断电保存变量.vi" "探头选择"() -> (w558:T5)
        n414 = Unbundle By Name(w558) -> ("DO探头选择"=w557:u16)
        n415 = case shown="2" w557 {
          tunnel: [w562 w563 w564] -> w556
          frame 0, Default {
            n416 = vi-ref "斯坦道多参数.lvlib:禹山溶解氧校准.vi"() -> (w562:refnum<vi>)
          }
          frame 1 {
            n417 = vi-ref "斯坦道多参数.lvlib:溶解氧电极校准.vi"() -> (w563:refnum<vi>)
          }
          frame 2 {
            n418 = vi-ref "斯坦道多参数.lvlib:纳清DO电极校准.vi"() -> (w564:refnum<vi>)
          }
        }
        n419 = property class="VI"(reference=w556) -> (reference out=w560:refnum<vi>, "Exec.State"=w559:T7)  [unwired: 1 in, 1 out]
        n420 = case shown="\"Bad\", 默认" w559 {
          tunnel: [w565 w567] -> w553
          tunnel: w560 -> [w565 w566]
          frame "Bad", Default {
          }
          frame "Idle" {
            n421 = invoke class="VI" method="Run VI"(reference=w566, "Wait until done"=FALSE ("结束前等待"), "Auto Dispose Ref"=FALSE ("自动销毁引用")) -> (reference out=w567:refnum<vi>)  [unwired: 2 in, 4 out]
          }
        }
        n422 = global read "多参数全局变量.vi" "校准VI引用句柄"() -> (w555:T13)
        n423 = invoke on="探头校准子面板" class="SubPnl" method="Remove VI"() -> (error out=w561:errorcluster)  [unwired: 3 in, 2 out]
        n424 = invoke on="探头校准子面板" class="SubPnl" method="Insert VI"(error in=w561, "VI Ref"=w553) -> ()  [unwired: 2 in, 4 out]
        n425 = Bundle By Name(cluster=w555, "DO校准VI引用句柄"=w553) -> (w554:T13)
        n426 = global write "多参数全局变量.vi" "校准VI引用句柄"(w554) -> ()
      }
      event "校准选择.浊度校准": Value Change {
        n427 = event-data() -> ()  [unwired: 1 in, 6 out]
        n428 = global read "断电保存变量.vi" "探头选择"() -> (w575:T5)
        n429 = Unbundle By Name(w575) -> ("浊度探头选择"=w574:u16)
        n430 = case shown="2" w574 {
          tunnel: [w579 w580 w581] -> w573
          frame 0, Default {
            n431 = vi-ref "斯坦道多参数.lvlib:禹山浊度校准.vi"() -> (w579:refnum<vi>)
          }
          frame 1 {
            n432 = vi-ref "斯坦道多参数.lvlib:浊度电极校准.vi"() -> (w580:refnum<vi>)
          }
          frame 2 {
            n433 = vi-ref "斯坦道多参数.lvlib:纳清浊度电极校准.vi"() -> (w581:refnum<vi>)
          }
        }
        n434 = property class="VI"(reference=w573) -> (reference out=w577:refnum<vi>, "Exec.State"=w576:T7)  [unwired: 1 in, 1 out]
        n435 = case shown="\"Bad\", 默认" w576 {
          tunnel: [w582 w584] -> w570
          tunnel: w577 -> [w582 w583]
          frame "Bad", Default {
          }
          frame "Idle" {
            n436 = invoke class="VI" method="Run VI"(reference=w583, "Wait until done"=FALSE ("结束前等待"), "Auto Dispose Ref"=FALSE ("自动销毁引用")) -> (reference out=w584:refnum<vi>)  [unwired: 2 in, 4 out]
          }
        }
        n437 = global read "多参数全局变量.vi" "校准VI引用句柄"() -> (w572:T13)
        n438 = invoke on="探头校准子面板" class="SubPnl" method="Remove VI"() -> (error out=w578:errorcluster)  [unwired: 3 in, 2 out]
        n439 = invoke on="探头校准子面板" class="SubPnl" method="Insert VI"(error in=w578, "VI Ref"=w570) -> ()  [unwired: 2 in, 4 out]
        n440 = Bundle By Name(cluster=w572, "TURB校准VI引用句柄"=w570) -> (w571:T13)
        n441 = global write "多参数全局变量.vi" "校准VI引用句柄"(w571) -> ()
      }
      event "校准选择.叶绿素a校准": Value Change {
        n442 = event-data() -> ()  [unwired: 1 in, 6 out]
        n443 = global read "断电保存变量.vi" "探头选择"() -> (w591:T5)
        n444 = Unbundle By Name(w591) -> ("叶绿素a探头选择"=w590:u16)
        n445 = case shown="2" w590 {
          tunnel: [w596 _ w597] -> w592
          frame 0, Default {
            n446 = vi-ref "禹山叶绿素a校准.vi"() -> (w596:refnum<vi>)
          }
          frame 1 {
          }
          frame 2 {
            n447 = vi-ref "斯坦道多参数.lvlib:纳清叶绿素a电极校准.vi"() -> (w597:refnum<vi>)
          }
        }
        n448 = property class="VI"(reference=w592) -> (reference out=w594:refnum<vi>, "Exec.State"=w593:T7)  [unwired: 1 in, 1 out]
        n449 = case shown="\"Bad\", 默认" w593 {
          tunnel: [w598 w600] -> w587
          tunnel: w594 -> [w598 w599]
          frame "Bad", Default {
          }
          frame "Idle" {
            n450 = invoke class="VI" method="Run VI"(reference=w599, "Wait until done"=FALSE ("结束前等待"), "Auto Dispose Ref"=FALSE ("自动销毁引用")) -> (reference out=w600:refnum<vi>)  [unwired: 2 in, 4 out]
          }
        }
        n451 = global read "多参数全局变量.vi" "校准VI引用句柄"() -> (w589:T13)
        n452 = invoke on="探头校准子面板" class="SubPnl" method="Remove VI"() -> (error out=w595:errorcluster)  [unwired: 3 in, 2 out]
        n453 = invoke on="探头校准子面板" class="SubPnl" method="Insert VI"(error in=w595, "VI Ref"=w587) -> ()  [unwired: 2 in, 4 out]
        n454 = Bundle By Name(cluster=w589, "CHLA校准VI引用句柄"=w587) -> (w588:T13)
        n455 = global write "多参数全局变量.vi" "校准VI引用句柄"(w588) -> ()
      }
      event "校准选择.藻密度校准": Value Change {
        n456 = event-data() -> ()  [unwired: 1 in, 6 out]
        n457 = global read "断电保存变量.vi" "探头选择"() -> (w607:T5)
        n458 = Unbundle By Name(w607) -> ("蓝绿藻探头选择"=w606:u16)
        n459 = case shown="2" w606 {
          tunnel: [_ w612] -> w608
          frame 0, Default {
          }
          frame 2 {
            n460 = vi-ref "斯坦道多参数.lvlib:纳清蓝绿藻电极校准.vi"() -> (w612:refnum<vi>)
          }
        }
        n461 = property class="VI"(reference=w608) -> (reference out=w610:refnum<vi>, "Exec.State"=w609:T7)  [unwired: 1 in, 1 out]
        n462 = case shown="\"Bad\", 默认" w609 {
          tunnel: [w613 w615] -> w603
          tunnel: w610 -> [w613 w614]
          frame "Bad", Default {
          }
          frame "Idle" {
            n463 = invoke class="VI" method="Run VI"(reference=w614, "Wait until done"=FALSE ("结束前等待"), "Auto Dispose Ref"=FALSE ("自动销毁引用")) -> (reference out=w615:refnum<vi>)  [unwired: 2 in, 4 out]
          }
        }
        n464 = global read "多参数全局变量.vi" "校准VI引用句柄"() -> (w605:T13)
        n465 = invoke on="探头校准子面板" class="SubPnl" method="Remove VI"() -> (error out=w611:errorcluster)  [unwired: 3 in, 2 out]
        n466 = invoke on="探头校准子面板" class="SubPnl" method="Insert VI"(error in=w611, "VI Ref"=w603) -> ()  [unwired: 2 in, 4 out]
        n467 = Bundle By Name(cluster=w605, "BGA校准VI引用句柄"=w603) -> (w604:T13)
        n468 = global write "多参数全局变量.vi" "校准VI引用句柄"(w604) -> ()
      }
      event "校准选择.ORP校准": Value Change {
        n469 = event-data() -> ()  [unwired: 1 in, 6 out]
        n470 = global read "断电保存变量.vi" "探头选择"() -> (w622:T5)
        n471 = Unbundle By Name(w622) -> ("orp探头选择"=w621:u16)
        n472 = case shown="1" w621 {
          tunnel: [_ w627] -> w623
          frame 0, Default {
          }
          frame 1 {
            n473 = vi-ref "斯坦道多参数.lvlib:ORP电极校准.vi"() -> (w627:refnum<vi>)
          }
        }
        n474 = property class="VI"(reference=w623) -> (reference out=w625:refnum<vi>, "Exec.State"=w624:T7)  [unwired: 1 in, 1 out]
        n475 = case shown="\"Bad\", 默认" w624 {
          tunnel: [w628 w630] -> w618
          tunnel: w625 -> [w628 w629]
          frame "Bad", Default {
          }
          frame "Idle" {
            n476 = invoke class="VI" method="Run VI"(reference=w629, "Wait until done"=FALSE ("结束前等待"), "Auto Dispose Ref"=FALSE ("自动销毁引用")) -> (reference out=w630:refnum<vi>)  [unwired: 2 in, 4 out]
          }
        }
        n477 = global read "多参数全局变量.vi" "校准VI引用句柄"() -> (w620:T13)
        n478 = invoke on="探头校准子面板" class="SubPnl" method="Remove VI"() -> (error out=w626:errorcluster)  [unwired: 3 in, 2 out]
        n479 = Bundle By Name(cluster=w620, "ORP校准VI引用句柄"=w618) -> (w619:T13)
        n480 = invoke on="探头校准子面板" class="SubPnl" method="Insert VI"(error in=w626, "VI Ref"=w618) -> ()  [unwired: 2 in, 4 out]
        n481 = global write "多参数全局变量.vi" "校准VI引用句柄"(w619) -> ()
      }
    }
  }
  n482 = property on="编号" class="Str"("Visible"=w23) -> ()  [unwired: 2 in, 2 out]
  n483 = while {
    tunnel: [w640] -> _
    shift-right: [w638] -> _
    shift-left: w2 -> [w637]
    tunnel: w1 -> [w634]
    stop <- FALSE stop-if-true
    n484 = Wait (ms)(milliseconds to wait=u32 1000 ("等待时间（毫秒）")) -> ()  [unwired: 1 out]
    n485 = global read "多参数全局变量.vi" "配置文件 path"() -> (w633:path)
    n486 = Read from Text File(file (use dialog)=w633, error in=w634) -> (text=w638:string, error out=w635:errorcluster)  [unwired: 2 in, 2 out]
    n487 = Not Equal?(x=w638, y=w637) -> (x != y?=w636:bool)
    n488 = case shown="真" w636 {
      tunnel: [w642 w646] -> w640
      tunnel: w633 -> [_ w645]
      tunnel: w635 -> [w642 w644]
      frame False {
      }
      frame True {
        # "文件发生改变进行更新"
        n489 = call <vilib>:"Open Config Data.vi"("error in (no error)"=w644, "configuration file path"=w645) -> ("error out"=w650:errorcluster, "refnum"=w649:T12)  [unwired: 7 in, 1 out]
        n490 = vi-ref "断电保存变量.vi"() -> (w643:refnum<vi>)
        n491 = call <userlib>:"Read Panel from INI__ogtk.vi"("error in (no error)"=w650, "VI ref"=w643, "refnum"=w649) -> ("error out"=w648:errorcluster, "refnum out"=w647:T12)  [unwired: 7 in]
        n492 = call <vilib>:"Close Config Data.vi"("error in (no error)"=w648, "refnum"=w647) -> ("error out"=w646:errorcluster)  [unwired: 8 in, 1 out]
      }
    }
  }
  n493 = while {
    tunnel: w50 -> [w652]
    tunnel: w1 -> [_]
    stop <- FALSE stop-if-true
    n494 = Dequeue Element(queue=w652) -> (element=w651:string)  [unwired: 2 in, 3 out]
    n495 = case shown="\"open\"" w651 {
      tunnel: [_ w654 w664] -> _
      frame "假", Default {
      }
      frame "open" {
        n496 = global read "多参数全局变量.vi" "MB session in"() -> (w659:refnum<class "MB_Master.lvclass">)
        n497 = global read "断电保存变量.vi" "VISA资源名称"() -> (w661:refnum<visa-resource-name>)
        n498 = global read "断电保存变量.vi" "连接方式"() -> (w657:u16)
        n499 = call "close MB.vi"("MB session in"=w659) -> ("error out"=w662:errorcluster)  [unwired: 10 in]
        n500 = global read "断电保存变量.vi" "Port"() -> (w655:u16)
        n501 = global read "断电保存变量.vi" "IP"() -> (w656:string)
        n502 = call "open MB.vi"("Port (502)"=w655, "IP Address"=w656, "MODE"=w657, "error in (no error)"=w662, "Serial Config"=T15 {"baud rate (bps)"=9600, "stop bits"=10, "parity"=0, "flow control"=0, "timeout"=1000, "retries"=1}, "VISA资源名称"=w661) -> ("error out"=w654:errorcluster, "MB session out"=w658:refnum<class "MB_Master.lvclass">)  [unwired: 4 in]
        n503 = global write "多参数全局变量.vi" "MB session in"(w658) -> ()
      }
      frame "close" {
        n504 = global read "多参数全局变量.vi" "MB session in"() -> (w663:refnum<class "MB_Master.lvclass">)
        n505 = call "close MB.vi"("MB session in"=w663) -> ("error out"=w664:errorcluster)  [unwired: 10 in]
      }
    }
  }
  n506 = while {
    tunnel: w50 -> [w666]
    stop <- FALSE stop-if-true
    # "断线重连"
    n507 = global read "断电保存变量.vi" "连接方式"() -> (w667:u16)
    n508 = Wait (ms)(milliseconds to wait=u32 10000 ("等待时间（毫秒）")) -> ()  [unwired: 1 out]
    n509 = case shown="1" w667 {
      tunnel: w666 -> [_ w670]
      frame 0, Default {
      }
      frame 1 {
        n510 = case shown="真" "自动断线重连" {
          tunnel: w670 -> [_ w673]
          frame False {
          }
          frame True {
            n511 = global read "多参数全局变量.vi" "MB session in"() -> (w672:refnum<class "MB_Master.lvclass">)
            n512 = property class="MB_Master"(reference=w672) -> ("Properties:Session Valid"=w671:bool)  [unwired: 1 in, 2 out]
            n513 = case shown="假" w671 {
              tunnel: w673 -> [w674 _]
              frame False {
                n514 = Flush Queue(queue=w674) -> (queue out=w676:refnum<queue>)  [unwired: 1 in, 2 out]
                n515 = Enqueue Element(queue=w676, element="open" ("元素")) -> ()  [unwired: 2 in, 3 out]
              }
              frame True {
              }
            }
          }
        }
      }
    }
  }
